vi "Aim_And_Range.vi"() -> ()   [LabVIEW 2019]
uses:
  <vilib>/Rock Robotics/WPI/Joystick/XBox Buttons Indexer.ctl
  <vilib>/Rock Robotics/WPI/Joystick/XBox Axes Indexer.ctl
  <vilib>/Rock Robotics/WPI/ThirdParty/JAS_Junk/TrajLib/PIDController_AtSetpoint.vi
  <vilib>/Rock Robotics/WPI/ThirdParty/JAS_Junk/TrajLib/PIDController_SetPIDF.vi
  <vilib>/Rock Robotics/WPI/ThirdParty/JAS_Junk/TrajLib/PIDController_SetDerivativeFilter.vi
  <vilib>/Rock Robotics/WPI/ThirdParty/JAS_Junk/TrajLib/PIDController_SetIntegratorRange.vi
  <vilib>/Rock Robotics/WPI/ThirdParty/JAS_Junk/TrajLib/PIDController_SetTolerancePandV.vi
  <vilib>/Rock Robotics/WPI/ThirdParty/JAS_Junk/TrajLib/PIDController_DisableContinousInput.vi
  <vilib>/Rock Robotics/WPI/ThirdParty/JAS_Junk/TrajLib/PIDController_EnableContinousInput.vi
  <vilib>/Rock Robotics/WPI/ThirdParty/JAS_Junk/TrajLib/PIDController_Reset.vi
  <vilib>/Rock Robotics/WPI/ThirdParty/JAS_Junk/TrajLib/PIDController_New.vi
  <vilib>/Rock Robotics/WPI/ThirdParty/JAS_Junk/TrajLib/PIDController_SetOutputLimits.vi
  <vilib>/Rock Robotics/WPI/ThirdParty/JAS_Junk/TrajLib/PIDController_NewPeriod.vi
  <vilib>/Rock Robotics/SystemInterfaces/NetworkCommunication/NetComm_UsageReport_report.vi
  <vilib>/Rock Robotics/WPI/Utilities/WPI_GetSetVariantRefNum.vi
  <vilib>/Rock Robotics/Network Tables/NT Write Boolean.vi
  <vilib>/Rock Robotics/WPI/Joystick/WPI_JoystickArcadeMapping.vi
  <vilib>/Rock Robotics/Network Tables/NT Write Number.vi
  <vilib>/Rock Robotics/WPI/ThirdParty/JAS_Junk/TrajLib/Util_LibraryGlobals.vi
  <vilib>/Rock Robotics/WPI/ThirdParty/JAS_Junk/TrajLib/PIDController_AdvCalculate_FF_Sp_Pv.vi
  <vilib>/Rock Robotics/Network Tables/NT Write Numeric Array.vi
  <vilib>/Rock Robotics/WPI/ThirdParty/PhotonVisionLib/PhotonVisionLib.lvlib
  <vilib>/Rock Robotics/WPI/ThirdParty/JAS_Junk/TrajLib/Trajectory_Library.lvlib
panel:
  in  "Fiiducial ID":i32
  in  "Use Fiducial\nID":bool
  out "Auto Aim\nSelected":bool
  out "TargetFound":bool
  out "Yaw":dbl
  out "DistanceToTarget Meters":dbl
  out "Right Motor Demand":dbl format="%14.4f"
  out "Left Motor Demand":dbl format="%14.4f"
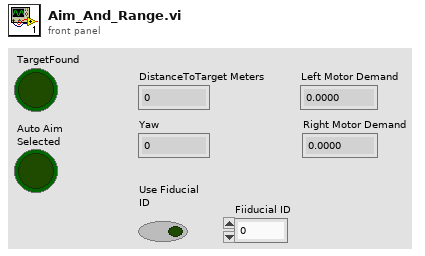
[diagram p1: front panel]
types:
  T1 = typedef "XBox Axes Indexer.ctl" = enum16{"Left X", "Left Y", "Left Trigger", "Right Trigger", "Right X", "Right Y"}
  T2 = typedef "XBox Buttons Indexer.ctl" = enum16{"A", "B", "X", "Y", "Left Bumper", "Right Bumper", "Back", "Start", "Left Joystick", "Right Joystick"}
  T3 = typedef "WPI_JoystickDevRef.ctl" = cluster{"Device":T4}
  T4 = typedef "WPI_JoystickDeviceEnum.ctl" = enum16{"USB 0", "USB 1", "USB 2", "USB 3", "USB 4", "USB 5"}
  T5 = typedef "WPI_RobotDriveDevRef.ctl" = cluster{"DevStatus":errorcluster, "Motors[]":T6[], "Square Inputs":bool, "Max Output":dbl}
  T6 = typedef "WPI_MotorControlDeviceRef.ctl" = cluster{"DeviceStatus":errorcluster, "Type":T7, "PWM":cluster{"PWM Channel":T8, "DeadBand":T9}, "CAN":cluster{"Device Number":u8, "SetOutput VI Ref":variant, "GetOutput VI Ref":variant, "Enable VI Ref":variant, "Disable VI Ref":variant, "Data":variant}, "Invert":bool, "DIO PWM":cluster{"PWM \"Enable\" Channel":T8, "DIOChannel":T10, "PWM Rate":dbl}}
  T7 = typedef "WPI_MotorControlType.ctl" = enum16{"PWM", "CAN", "DIO PWM"}
  T8 = typedef "FPGA_DIOPWMChannel.ctl" = enum8{"PWM 0", "PWM 1", "PWM 2", "PWM 3", "PWM 4", "PWM 5", "PWM 6", "PWM 7", "PWM 8", "PWM 9", "PWM MXP 0", "PWM MXP 1", "PWM MXP 2", "PWM MXP 3", "PWM MXP 4", "PWM MXP 5", "PWM MXP 6", "PWM MXP 7", "PWM MXP 8", "PWM MXP 9", "Invalid"}
  T9 = typedef "WPI_PWMDeadband.ctl" = cluster{"Name":string, "maxPositivePwm":i32, "minPositivePwm":i32, "centerPwm":i32, "maxNegativePwm":i32, "minNegativePwm":i32, "angularRange":u16}
  T10 = typedef "FPGA_DIOChannel.ctl" = enum8{"DIO 0", "DIO 1", "DIO 2", "DIO 3", "DIO 4", "DIO 5", "DIO 6", "DIO 7", "DIO 8", "DIO 9", "DIO MXP 0", "DIO MXP 1", "DIO MXP 2", "DIO MXP 3", "DIO MXP 4", "DIO MXP 5", "DIO MXP 6", "DIO MXP 7", "DIO MXP 8", "DIO MXP 9", "DIO MXP 10", "DIO MXP 11", "DIO MXP 12", "DIO MXP 13", "DIO MXP 14", "DIO MXP 15", "SPI Port CS1", "SPI Port CS2", "SPI Port CS3", "SPI Port MISO", "SPI Port MOSI", "Invalid"}
  T11 = typedef "PhotonVisionLib.lvlib/PhotonPipelineResultType.ctl" = cluster{"TargetCount":i32, "Latency_MilliSec":dbl, "Targets":T12[], "TimeStampSec":dbl}
  T12 = typedef "PhotonVisionLib.lvlib/PhotonTrackedTargetType.ctl" = cluster{"Yaw":dbl, "Pitch":dbl, "Area":dbl, "Skew":dbl, "MinAreaRectCorners":T13[], "BestCameraToTarget":T14, "FiiducialId":i32, "AltCameraToTarget":T14, "PoseAmbiguity":dbl, "DetectedCorners":T13[]}
  T13 = typedef "PhotonVisionLib.lvlib/TargetCornerType.ctl" = cluster{"X":dbl, "Y":dbl}
  T14 = typedef "Trajectory_Library.lvlib/TRANSFORM3D.ctl" = cluster{"TRANSLATION3D":T15, "ROTATION3D":T16, "XF":bool}
  T15 = typedef "Trajectory_Library.lvlib/TRANSLATION3D.ctl" = cluster{"X":dbl, "Y":dbl, "Z":dbl}
  T16 = typedef "Trajectory_Library.lvlib/ROTATION3D.ctl" = cluster{"Q_quaternion":T17}
  T17 = typedef "Trajectory_Library.lvlib/QUATERNION.ctl" = cluster{"R":dbl, "V":dbl[]}
  T18 = typedef "Trajectory_Library.lvlib/PID_ADV_LIMITS.ctl" = cluster{"MaxInput":dbl, "MinInput":dbl, "Continuous":bool, "MaxOutput":dbl, "MinOutput":dbl}
  T19 = typedef "Trajectory_Library.lvlib/PID_ADV_TUNING.ctl" = cluster{"Kf":dbl, "Kp":dbl, "Ki":dbl, "Kd":dbl, "MaximumIntegral":dbl, "MinimumIntegral":dbl, "Filter Derivative":bool}
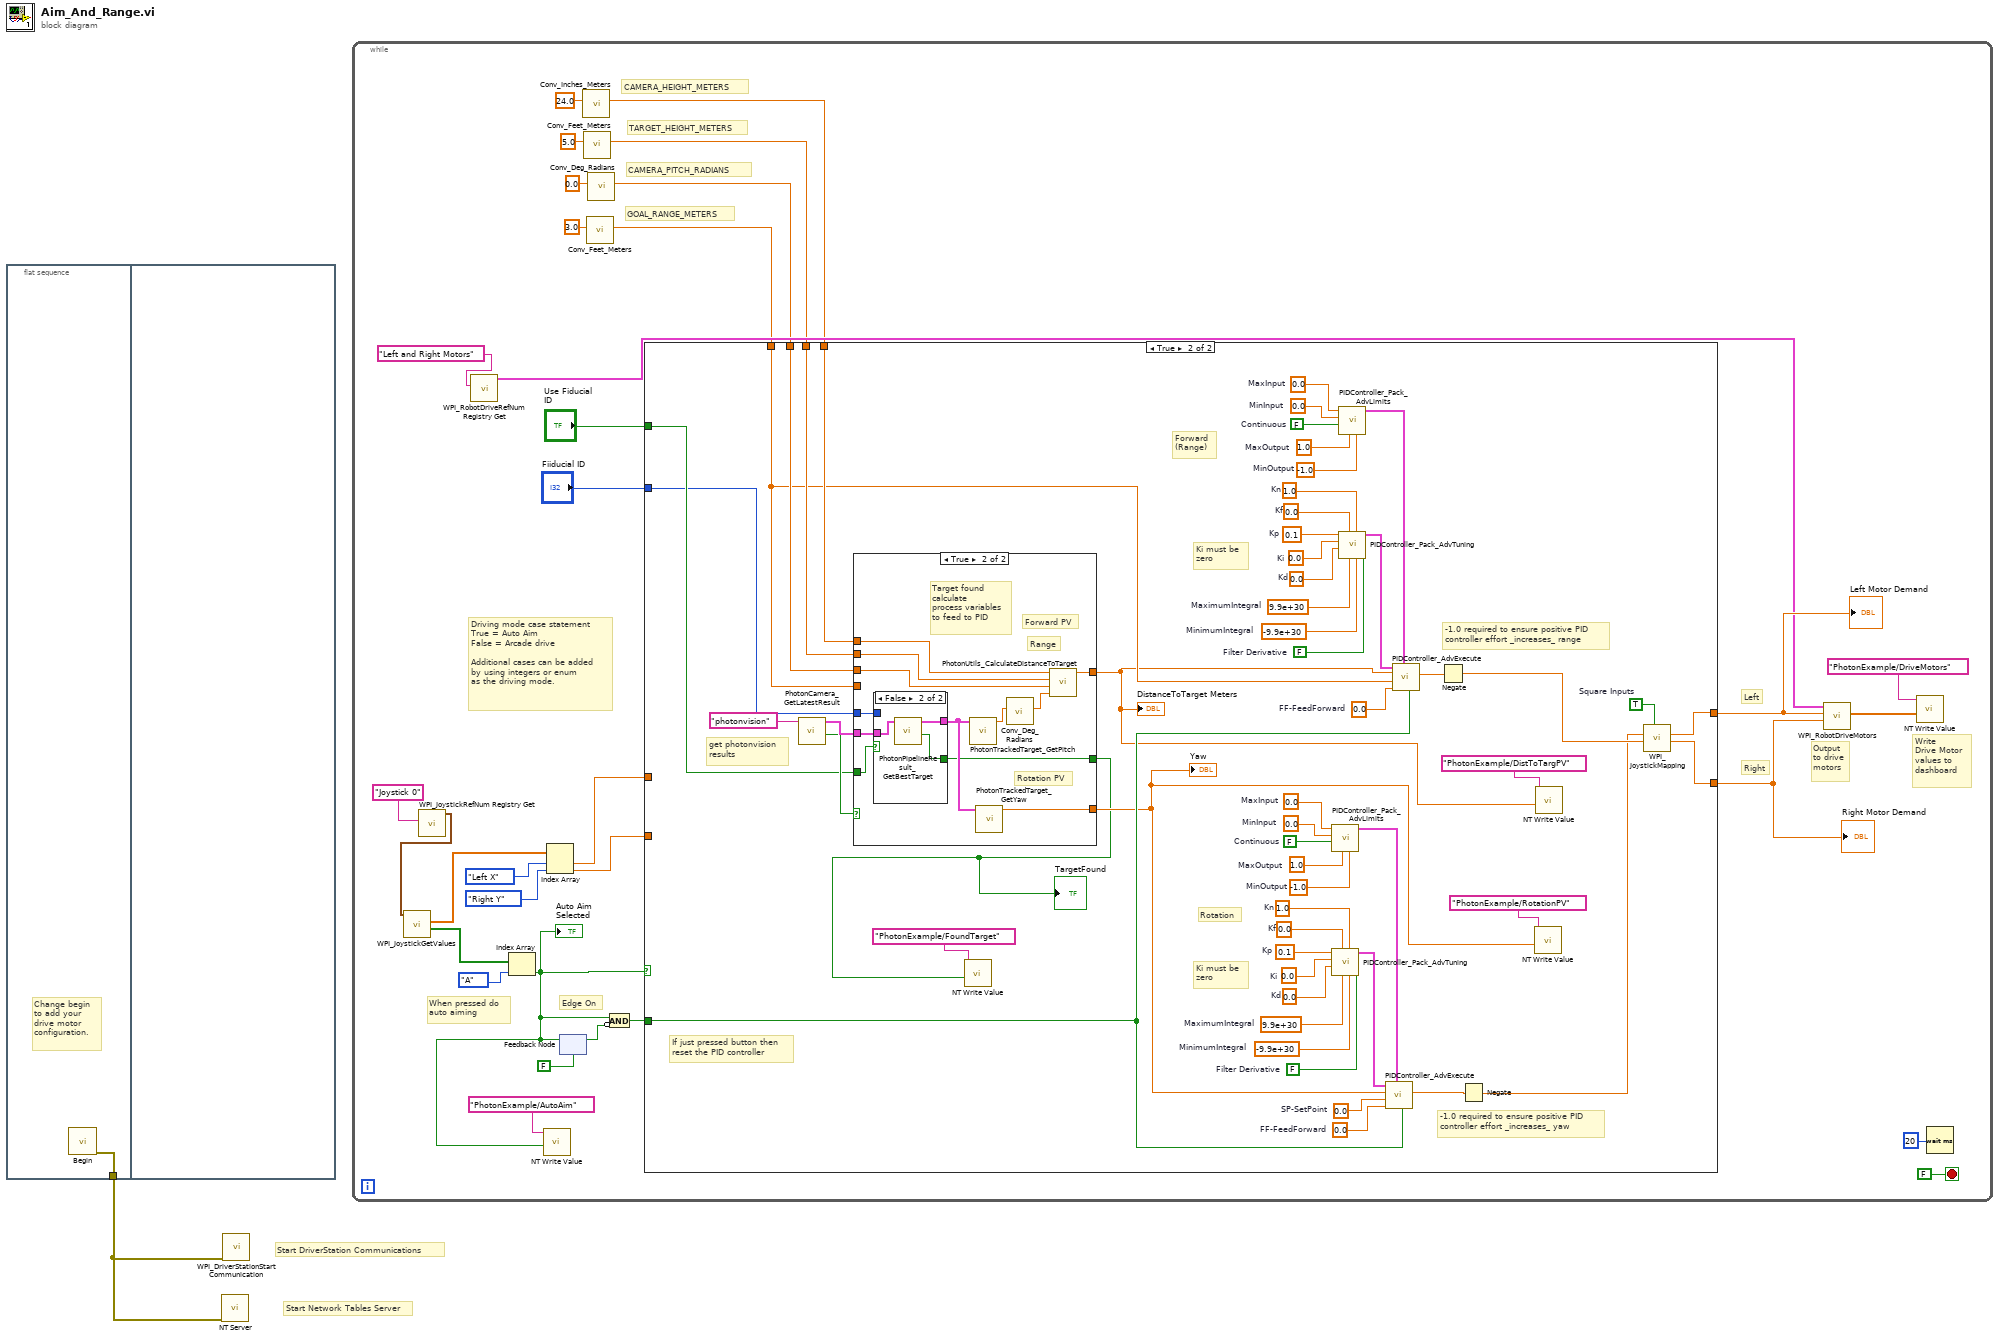
[diagram p0: block diagram]
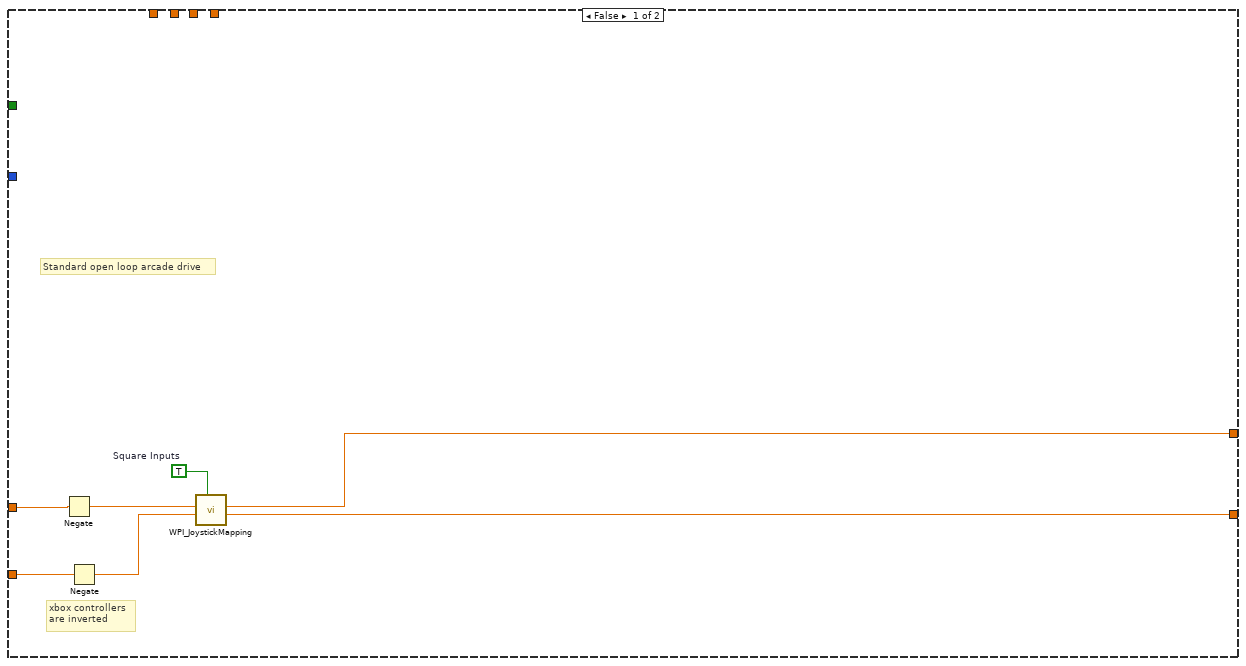
[diagram p2: hidden frame]
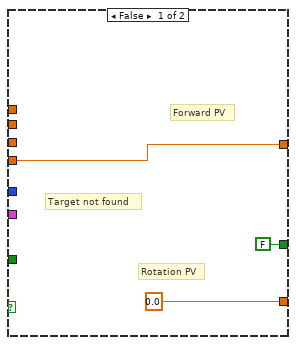
[diagram p3: hidden frame]
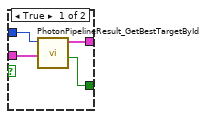
[diagram p4: hidden frame]
diagram:
  # "Start Network Tables Server"
  # "Start DriverStation Communications"
  n1 = flat-sequence {
    tunnel: [w2] -> w1
    frame #0 {
      # "Change begin\nto add your \ndrive motor\nconfiguration."
      n2 = call "Begin.vi"() -> ("error out"=w2:errorcluster)  [unwired: 11 in]
    }
    frame #1 {
    }
  }
  n3 = call <vilib>:"NT Server.vi"("error in (no error)"=w1) -> ()  [unwired: 11 in]
  n4 = call <vilib>:"WPI_DriverStationStart Communication.vi"("error in (no error)"=w1) -> ()  [unwired: 11 in]
  n5 = while {
    stop <- FALSE stop-if-true
    # "GOAL_RANGE_METERS"
    # "CAMERA_PITCH_RADIANS"
    # "TARGET_HEIGHT_METERS"
    # "CAMERA_HEIGHT_METERS"
    # "Write \nDrive Motor\nvalues to \ndashboard"
    # "Output\nto drive\nmotors"
    # "Edge On"
    # "Right"
    # "Left"
    # "Driving mode case statement\nTrue = Auto Aim\nFalse = Arcade drive\n\nAdditional cases can be added\nby using integers or enum\nas the driving mode."
    # "When pressed do\nauto aiming"
    n6 = call <vilib>:"WPI_JoystickRefNum Registry Get.vi"("refnum name"="Joystick 0") -> ("JoystickDevRef"=w13:T3)  [unwired: 9 in, 1 out]
    n7 = call <vilib>:"WPI_JoystickGetValues.vi"("JoystickDevRef"=w13) -> ("Buttons"=w33:bool[], "Axes"=w32:dbl[])  [unwired: 6 in, 3 out]
    n8 = call <vilib>:"WPI_RobotDriveRefNum Registry Get.vi"("refnum name"="Left and Right Motors") -> ("RobotDriveDevRef"=w11:T5)  [unwired: 9 in, 1 out]
    n9 = Index Array(array=w33, index=XBox_Buttons_Indexer."A" ("XBox Buttons")) -> (element=w17:bool)
    "Auto Aim\nSelected" <- w17
    n10 = call-poly <vilib>:"NT Write Value.vi"("Boolean"=w17, "Name"="PhotonExample/AutoAim") -> ()  [unwired: 9 in, 1 out]
    n11 = Index Array(array=w32, index #1=XBox_Axes_Indexer."Left X" ("XBox Axes"), index #2=XBox_Axes_Indexer."Right Y" ("XBox Axes")) -> (element #1=w28:dbl, element #2=w27:dbl)
    n12 = feedback-in #1(w17) -> ()
    n13 = feedback #1(FALSE) -> (w24:bool)
    n14 = call <vilib>:"Conv_Inches_Meters.vi"("INCH"=24.0) -> ("Meters"=w3:dbl)  [unwired: 10 in]
    n15 = call <vilib>:"Conv_Feet_Meters.vi"("Feet"=5.0) -> ("Meters"=w4:dbl)  [unwired: 10 in]
    n16 = call <vilib>:"Conv_Feet_Meters.vi"("Feet"=3.0) -> ("Meters"=w6:dbl)  [unwired: 10 in]
    n17 = call <vilib>:"Conv_Deg_Radians.vi"("Degress"=0.0) -> ("Radians"=w5:dbl)  [unwired: 10 in]
    n18 = Compound Arithmetic op=AND(w17, invert w24) -> (w25:bool)
    n19 = case shown="True" w17 {
      tunnel: w28 -> [w41 _]
      tunnel: w27 -> [w40 _]
      tunnel: [w36 w95] -> w26
      tunnel: [w35 w94] -> w19
      tunnel: w25 -> [_ w61]
      tunnel: w3 -> [_ w58]
      tunnel: w4 -> [_ w57]
      tunnel: w5 -> [_ w56]
      tunnel: w6 -> [_ w55]
      tunnel: "Use Fiducial\nID" -> [_ w44]
      tunnel: "Fiiducial ID" -> [_ w43]
      frame False {
        w37 = TRUE  # Square Inputs
        # "Standard open loop arcade drive"
        # "xbox controllers\nare inverted"
        n20 = Negate(x=w41) -> (-x=w39:dbl)
        n21 = Negate(x=w40) -> (-x=w38:dbl)
        n22 = call-poly <vilib>:"WPI_JoystickMapping.vi"("Square Inputs"=w37, "Y axis value"=w38, "X axis value"=w39) -> ("Right Motor Value"=w35:dbl, "Left Motor Value"=w36:dbl)  [unwired: 7 in]
      }
      frame True {
        w59 = 0.0  # FF-FeedForward
        w60 = 0.0  # FF-FeedForward
        w62 = 0.0  # SP-SetPoint
        w78 = 1.0  # Kn
        w77 = 0.1  # Kp
        w76 = 0.0  # Ki
        w75 = 0.0  # Kd
        w74 = 0.0  # Kf
        w73 = 9.9e+30  # MaximumIntegral
        w72 = -9.9e+30  # MinimumIntegral
        w71 = FALSE  # Filter Derivative
        w69 = 0.0  # MinInput
        w68 = FALSE  # Continuous
        w67 = 1.0  # MaxOutput
        w70 = -1.0  # MinOutput
        w66 = 0.0  # MaxInput
        w93 = 1.0  # Kn
        w92 = 0.1  # Kp
        w91 = 0.0  # Ki
        w90 = 0.0  # Kd
        w89 = 0.0  # Kf
        w88 = 9.9e+30  # MaximumIntegral
        w87 = -9.9e+30  # MinimumIntegral
        w86 = FALSE  # Filter Derivative
        w84 = 0.0  # MinInput
        w83 = FALSE  # Continuous
        w82 = 1.0  # MaxOutput
        w85 = -1.0  # MinOutput
        w81 = 0.0  # MaxInput
        w96 = TRUE  # Square Inputs
        # "-1.0 required to ensure positive PID \ncontroller effort _increases_ range"
        # "-1.0 required to ensure positive PID \ncontroller effort _increases_ yaw"
        # "Ki must be \nzero"
        # "Ki must be \nzero"
        # "If just pressed button then\nreset the PID controller"
        # "Rotation"
        # "Forward \n(Range)"
        # "get photonvision\nresults"
        n23 = call <vilib>:"PhotonCamera_GetLatestResult.vi"("CameraName"="photonvision") -> ("HasTargets"=w49:bool, "PipelineResult"=w63:T11)  [unwired: 9 in]
        n24 = case shown="True" w49 {
          tunnel: w63 -> [_ w112]
          tunnel: [w99 w108] -> w46
          tunnel: [0.0 w107] -> w45
          tunnel: w58 -> [_ w104]
          tunnel: w57 -> [_ w105]
          tunnel: w56 -> [_ w106]
          tunnel: w55 -> [w99 _]
          tunnel: w44 -> [_ w103]
          tunnel: [FALSE ("TargetFound") w102] -> w42
          tunnel: w43 -> [_ w101]
          frame False {
            # "Forward PV"
            # "Rotation PV"
            # "Target not found"
          }
          frame True {
            # "Target found\ncalculate\nprocess variables\nto feed to PID"
            # "Range"
            # "Forward PV"
            # "Rotation PV"
            n25 = case shown="False" w103 {
              tunnel: w112 -> [w114 w119]
              tunnel: [w116 w118] -> w109
              tunnel: [w115 w117] -> w102
              tunnel: w101 -> [w113 _]
              frame True {
                n26 = call <vilib>:"PhotonPipelineResult_GetBestTargetById.vi"("PhotonPipelineResult"=w114, "FiducialId"=w113) -> ("Target Found"=w115:bool, "PhotonTrackedTarget"=w116:T12)  [unwired: 7 in, 1 out]
              }
              frame False {
                n27 = call <vilib>:"PhotonPipelineResult_GetBestTarget.vi"("PhotonPipelineResult"=w119) -> ("TargetFound"=w117:bool, "PhotonTrackedTarget"=w118:T12)  [unwired: 9 in]
              }
            }
            n28 = call <vilib>:"PhotonTrackedTarget_GetPitch.vi"("TrackedTarget"=w109) -> ("Pitch"=w111:dbl)  [unwired: 10 in]
            n29 = call <vilib>:"PhotonTrackedTarget_GetYaw.vi"("TrackedTarget"=w109) -> ("Yaw"=w107:dbl)  [unwired: 10 in]
            n30 = call <vilib>:"Conv_Deg_Radians.vi"("Degress"=w111) -> ("Radians"=w110:dbl)  [unwired: 10 in]
            n31 = call <vilib>:"PhotonUtils_CalculateDistanceToTarget.vi"("TargetPitch_Radians"=w110, "CameraPitch_Radians"=w106, "TargetHeight_Meters"=w105, "CameraHeight_Meters"=w104) -> ("DistanceToTarget_Meters"=w108:dbl)  [unwired: 7 in]
          }
        }
        "DistanceToTarget Meters" <- w46
        "Yaw" <- w45
        "TargetFound" <- w42
        n32 = call-poly <vilib>:"NT Write Value.vi"("Boolean"=w42, "Name"="PhotonExample/FoundTarget") -> ()  [unwired: 9 in, 1 out]
        n33 = call <vilib>:"PIDController_Pack_AdvLimits.vi"("MinOutput"=w70, "MaxOutput"=w67, "Continuous"=w68, "MinInput"=w69, "MaxInput"=w66) -> ("Adv PID Limits"=w64:T18)  [unwired: 6 in]
        n34 = call <vilib>:"PIDController_Pack_AdvTuning.vi"("Filter Derivative"=w71, "MinimumIntegral"=w72, "Kn"=w78, "MaximumIntegral"=w73, "Kf"=w74, "Kd"=w75, "Ki"=w76, "Kp"=w77) -> ("Adv PID Tuning"=w65:T19)  [unwired: 3 in]
        n35 = call <vilib>:"PIDController_Pack_AdvLimits.vi"("MinOutput"=w85, "MaxOutput"=w82, "Continuous"=w83, "MinInput"=w84, "MaxInput"=w81) -> ("Adv PID Limits"=w79:T18)  [unwired: 6 in]
        n36 = call <vilib>:"PIDController_Pack_AdvTuning.vi"("Filter Derivative"=w86, "MinimumIntegral"=w87, "Kn"=w93, "MaximumIntegral"=w88, "Kf"=w89, "Kd"=w90, "Ki"=w91, "Kp"=w92) -> ("Adv PID Tuning"=w80:T19)  [unwired: 3 in]
        n37 = call <vilib>:"PIDController_AdvExecute.vi"("Reset"=w61, "Adv PID Limits"=w64, "FF-FeedForward"=w59, "SP-SetPoint"=w62, "PV-Measurement"=w45, "Adv PID Tuning"=w65) -> ("CO-ControlOutput"=w52:dbl)  [unwired: 3 in, 2 out]
        n38 = call <vilib>:"PIDController_AdvExecute.vi"("Reset"=w61, "Adv PID Limits"=w79, "FF-FeedForward"=w60, "SP-SetPoint"=w55, "PV-Measurement"=w46, "Adv PID Tuning"=w80) -> ("CO-ControlOutput"=w54:dbl)  [unwired: 3 in, 2 out]
        n39 = Negate(x=w54) -> (-x=w53:dbl)
        n40 = Negate(x=w52) -> (-x=w51:dbl)
        n41 = call-poly <vilib>:"NT Write Value.vi"("Numeric"=w45, "Name"="PhotonExample/RotationPV") -> ()  [unwired: 9 in, 1 out]
        n42 = call-poly <vilib>:"NT Write Value.vi"("Numeric"=w46, "Name"="PhotonExample/DistToTargPV") -> ()  [unwired: 9 in, 1 out]
        n43 = call-poly <vilib>:"WPI_JoystickMapping.vi"("Square Inputs"=w96, "Y axis value"=w53, "X axis value"=w51) -> ("Right Motor Value"=w94:dbl, "Left Motor Value"=w95:dbl)  [unwired: 7 in]
      }
    }
    "Left Motor Demand" <- w26
    "Right Motor Demand" <- w19
    n44 = call <vilib>:"WPI_RobotDriveMotors.vi"("RightSpeed"=w19, "LeftSpeed"=w26, "RobotDriveDevRef"=w11) -> ("Motor Values"=w21:dbl[])  [unwired: 6 in, 2 out]
    n45 = call-poly <vilib>:"NT Write Value.vi"("Numeric Array"=w21, "Name"="PhotonExample/DriveMotors") -> ()  [unwired: 9 in, 1 out]
    n46 = Wait (ms)(milliseconds to wait=u32 20) -> ()  [unwired: 1 out]
  }
